vi "onInterruptProcessTriggers.vi"(8 "error in (no error)":errorcluster, 10 "model in":refnum<class "IModel.lvclass">, 11 "EnabledState in":refnum<class "EnabledState.lvclass">) -> (0 "error out":errorcluster, 2 "model out":refnum<class "IModel.lvclass">, 3 "EnabledState out":refnum<class "EnabledState.lvclass">)   [LabVIEW 2016, in "States.lvlib" / "EnabledState.lvclass"]
uses:
  EnabledState.lvclass
  IModel/IModel.lvclass
  ts_sallv_exa/DataTypes/logevent_SummaryState.ctl
  ts_sallv_exa/SALLV_EXA.lvlib
  ts_sallv_exa/DataTypes/logevent_DetailedState.ctl
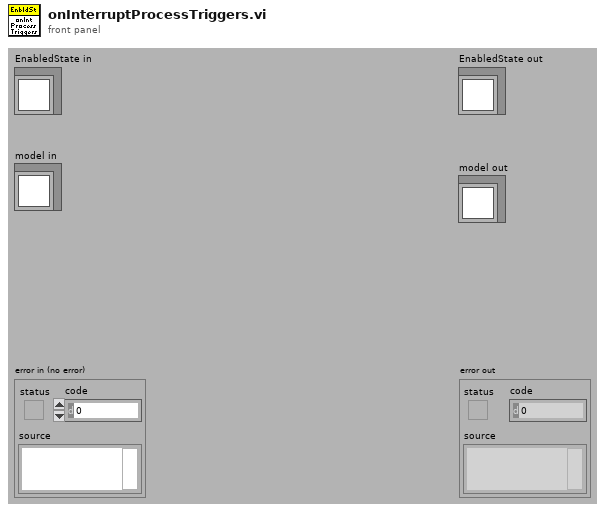
[diagram p1: front panel]
types:
  T1 = typedef "SALLV_EXA.lvlib/logevent_DetailedState.ctl" = cluster{"detailedState":enum16{"", " DisabledState", "EnabledState", "FaultState", "OfflineState", "StandbyState"}, "priority":i32}
  T2 = typedef "SALLV_EXA.lvlib/logevent_SummaryState.ctl" = cluster{"summaryState":enum16{"", " OfflineState", "StandbyState", "DisabledState", "EnabledState", "FaultState"}, "priority":i32}
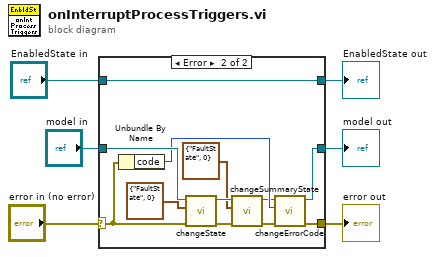
[diagram p0: block diagram]
diagram:
  n1 = case shown="Error" "error in (no error)" {
    selector: "error in (no error)" -> [w9 w16]
    tunnel: [w9 w13] -> w5
    tunnel: [w7 w17] -> w4
    tunnel: "model in" -> [w7 w21]
    tunnel: [w8 w12] -> w2
    tunnel: "EnabledState in" -> [w8 w12]
    frame No Error {
    }
    frame Error {
      n2 = Unbundle By Name(w16) -> ("code"=w19:i32)
      n3 = call-dynamic "changeState.vi"("error in (no error)"=w16, "DetailedState"=T1 {"detailedState"=enum."FaultState", "priority"=0} ("logevent_DetailedState"), "IModel in"=w21) -> ("error out"=w15:errorcluster, "IModel out"=w20:refnum<class "IModel.lvclass">)  [unwired: 7 in]
      n4 = call-dynamic "changeSummaryState.vi"("error in (no error)"=w15, "logevent_SummaryState"=T2 {"summaryState"=enum."FaultState", "priority"=0}, "IModel in"=w20) -> ("error out"=w14:errorcluster, "IModel out"=w18:refnum<class "IModel.lvclass">)  [unwired: 7 in]
      n5 = call-dynamic "changeErrorCode.vi"("error in (no error)"=w14, "error.code"=w19, "IModel in"=w18) -> ("error out"=w13:errorcluster, "IModel out"=w17:refnum<class "IModel.lvclass">)  [unwired: 7 in]
    }
  }
  "error out" <- w5
  "EnabledState out" <- w2
  "model out" <- w4
